vi "Read All Attributes.vi"(6 "error in (no error)":errorcluster, 9 "HDF5 Ref":T1) -> (0 "error out":errorcluster, 1 "Values":variant[](array[variant]), 2 "Names":string[](array[string]), 3 "HDF5 Ref out":T1)   [LabVIEW 2017]
doc: "Reads all attribute attached to the specified HDF5 object"
uses:
  <vilib>/UPVI/lvhdf5/library.llb/HDF5 Ref.ctl
panel:
  # "LVHDF5 Toolkit\nCopyright (c) 2005-2013 by Jason D. Sommerville\nCopyright (c) 2014 by UPVI, LLC.\n\nThis use and distribution of this file is governed by the terms found in \nLICENSE.txt distributed with this toolkit and installed at\n <user.lib>\\_lvhdf5\\LICENSE.txt"
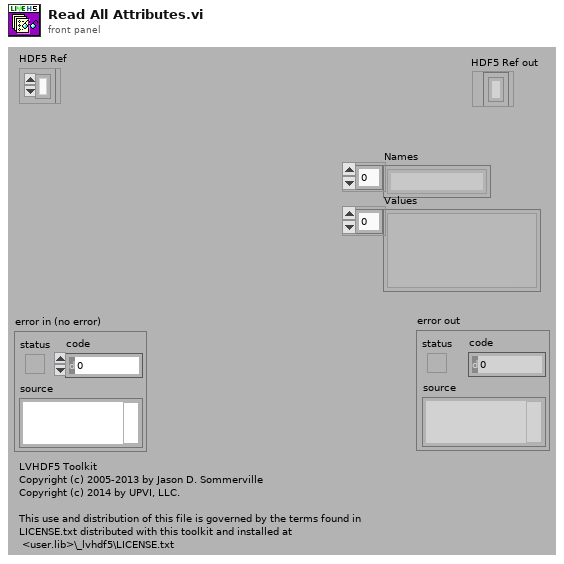
[diagram p1: front panel]
types:
  T1 = typedef "HDF5 Ref.ctl" = refnum<k1>
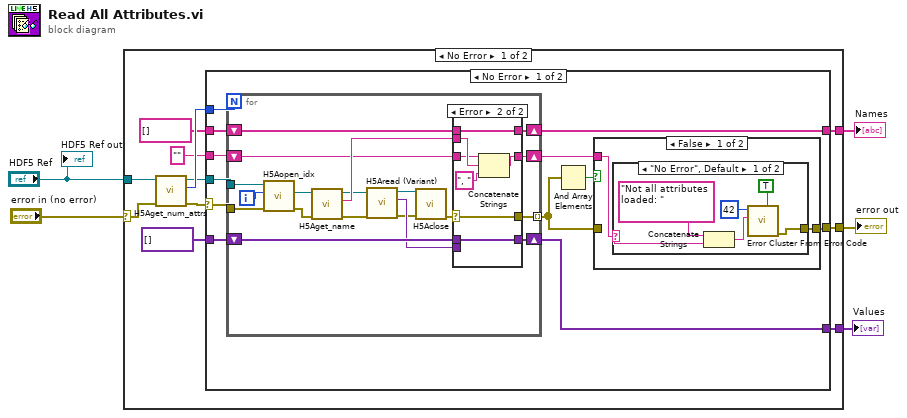
[diagram p0: block diagram]
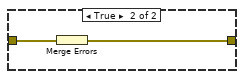
[diagram p3: hidden frame]
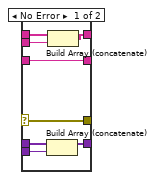
[diagram p4: hidden frame]
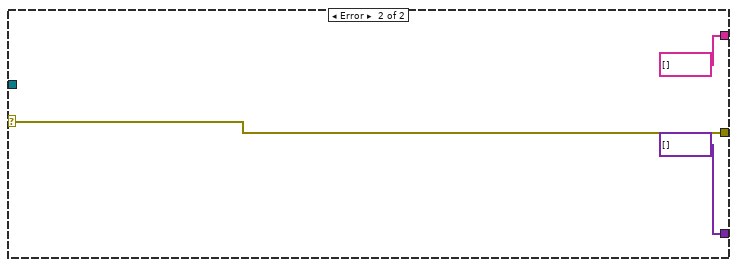
[diagram p6: hidden frame]
diagram:
  n1 = case shown="No Error" "error in (no error)" {
    selector: "error in (no error)" -> [w15 w76]
    tunnel: [w6 w76] -> w4
    tunnel: "HDF5 Ref" -> [w16 _]
    tunnel: [w12 string[] []] -> w2
    tunnel: [w11 variant[] []] -> w1
    frame No Error {
      n2 = call <vilib>:"H5Aget_num_attrs.vi"("error in (no error)"=w15, "HDF5 Ref"=w16) -> ("error out"=w10:errorcluster, "Number of Attributes"=w14:i32, "HDF5 Ref out"=w13:T1)  [unwired: 5 in]
      n3 = case shown="No Error" w10 {
        selector: w10 -> [w24 w73]
        tunnel: w14 -> [w28 _]
        tunnel: w13 -> [w27 _]
        tunnel: [w26 _] -> w12
        tunnel: [w25 _] -> w11
        tunnel: string[] [] ("Names") -> [w23 _]
        tunnel: variant[] [] ("Values") -> [w22 _]
        tunnel: "" ("Name") -> [w21 _]
        tunnel: [w18 w73] -> w6
        frame No Error {
          n4 = for {
            N: w28 -> [_]
            tunnel: w27 -> [w56]
            tunnel: w24 -> [w55]
            shift-right: [w42] -> w26
            shift-left: w23 -> [w54]
            shift-right: [w51] -> w25
            shift-left: w22 -> [w52]
            shift-right: [w40] -> w19
            shift-left: w21 -> [w41]
            tunnel: [w39] -> w17 mode=indexing
            i -> [w57]
            n5 = call <vilib>:"H5Aopen_idx.vi"("error in (no error)"=w55, "Index"=w57, "HDF5 Ref"=w56) -> ("error out"=w47:errorcluster, "HDF5 Attr Ref"=w49:T1)  [unwired: 4 in, 1 out]
            n6 = call <vilib>:"H5Aget_name.vi"("error in (no error)"=w47, "HDF5 Attr Ref"=w49) -> ("error out"=w46:errorcluster, "Name"=w53:string, "HDF5 Attr Ref out"=w48:T1)  [unwired: 5 in]
            n7 = call <vilib>:"H5Aread (Variant).vi"("error in (no error)"=w46, "HDF5 Attr Ref"=w48) -> ("error out"=w45:errorcluster, "Data out"=w50:variant, "HDF5 Attr Ref out"=w44:T1)  [unwired: 5 in]
            n8 = call <vilib>:"H5Aclose.vi"("error in (no error)"=w45, "HDF5 Dataset Ref"=w44) -> ("error out"=w43:errorcluster)  [unwired: 7 in]
            n9 = case shown="Error" w43 {
              selector: w43 -> [w58 w66]
              tunnel: w54 -> [w65 w72]
              tunnel: w53 -> [w60 w69]
              tunnel: w52 -> [w64 w71]
              tunnel: [w63 w71] -> w51
              tunnel: w50 -> [w62 _]
              tunnel: [w61 w72] -> w42
              tunnel: w41 -> [w59 w68]
              tunnel: [w59 w67] -> w40
              tunnel: [w58 w66] -> w39
              frame No Error {
                n10 = Build Array (concatenate)(w64, w62) -> (w63:variant[])
                n11 = Build Array (concatenate)(w65, w60) -> (w61:string[])
              }
              frame Error {
                n12 = Concatenate Strings(w68, w69, ", " ("string")) -> (w67:string)
              }
            }
          }
          n13 = And Array Elements(Boolean array=w17) -> (logical AND=w20:bool)
          n14 = case shown="False" w20 {
            tunnel: [w30 w37] -> w18
            tunnel: w17 -> [_ w38]
            tunnel: w19 -> [w29 _]
            frame False {
              n15 = case shown="\"No Error\", Default" w29 {
                selector: w29 -> [w33 _]
                tunnel: [w31 _] -> w30
                frame "No Error", Default {
                  n16 = Concatenate Strings("Not all attributes loaded: " ("string"), w33) -> (w32:string)
                  n17 = call <vilib>:"Error Cluster From Error Code.vi"("is warning? (False)"=TRUE, "error message (\"\")"=w32, "error code (0)"=42) -> ("error out"=w31:errorcluster)  [unwired: 6 in]
                }
                frame "" {
                }
              }
            }
            frame True {
              n18 = Merge Errors(w38) -> (w37:errorcluster)
            }
          }
        }
        frame Error {
        }
      }
    }
    frame Error {
    }
  }
  "error out" <- w4
  "Names" <- w2
  "Values" <- w1
  "HDF5 Ref out" <- "HDF5 Ref"
